vi "Teleop.vi"(10 "Match Info":T1={"Autonomous Elapsed Seconds"=0.0, "TeleOp Elapsed Seconds"=0.0, "Disabled Elapsed Seconds"=0.0, "Visited Autonomous"=FALSE, "Visited TeleOp"=FALSE, "Visited Disabled"=FALSE, "Autonomous Settings"={"Autonomous Style"=enum."Independent", "VI Refnum"=refnum}}, 11 "Call Context":T2) -> ()   [LabVIEW 2017]
doc: "This VI is called for each enabled TeleOp packet received from the DS. It is typically used to read from joysticks and other inputs and update I/O or setpoints for timed control loops. It should complete and return within 20 milliseconds or risk missing DS packets."
uses:
  <vilib>/Rock Robotics/WPI/DriverStation/WPI_DriverStationDerivedRobotMode.ctl
  <vilib>/Rock Robotics/WPI/DriverStation/WPI_DriverStationMatch Info.ctl
  Framework/Robot Global Data.vi
panel:
  out "Hardware Fault":bool
  out "Temperature Fault":bool
  out "Battery Voltage Fault":bool
  out "Current Faults":bool[](array[boolean])
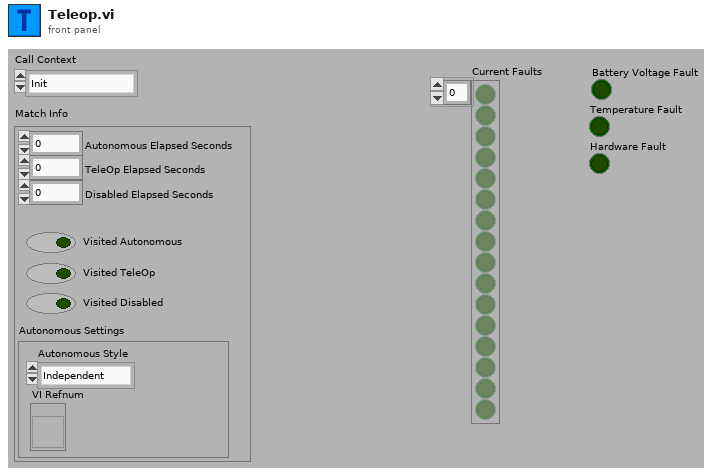
[diagram p1: front panel]
types:
  T1 = typedef "WPI_DriverStationMatch Info.ctl" = cluster{"Autonomous Elapsed Seconds":dbl, "TeleOp Elapsed Seconds":dbl, "Disabled Elapsed Seconds":dbl, "Visited Autonomous":bool, "Visited TeleOp":bool, "Visited Disabled":bool, "Autonomous Settings":cluster{"Autonomous Style":enum16{"Iterative", "Independent"}, "VI Refnum":refnum<vi>}}
  T2 = typedef "WPI_DriverStationDerivedRobotMode.ctl" = enum16{"Init", "Execute", "Stop"}
  T3 = enum16{"Linear", "Square  Root", "Square", "n^x"}
  T4 = enum16{"Normal", "Square", "Square with Rate", "Square Root", "Linear", "Exponential"}
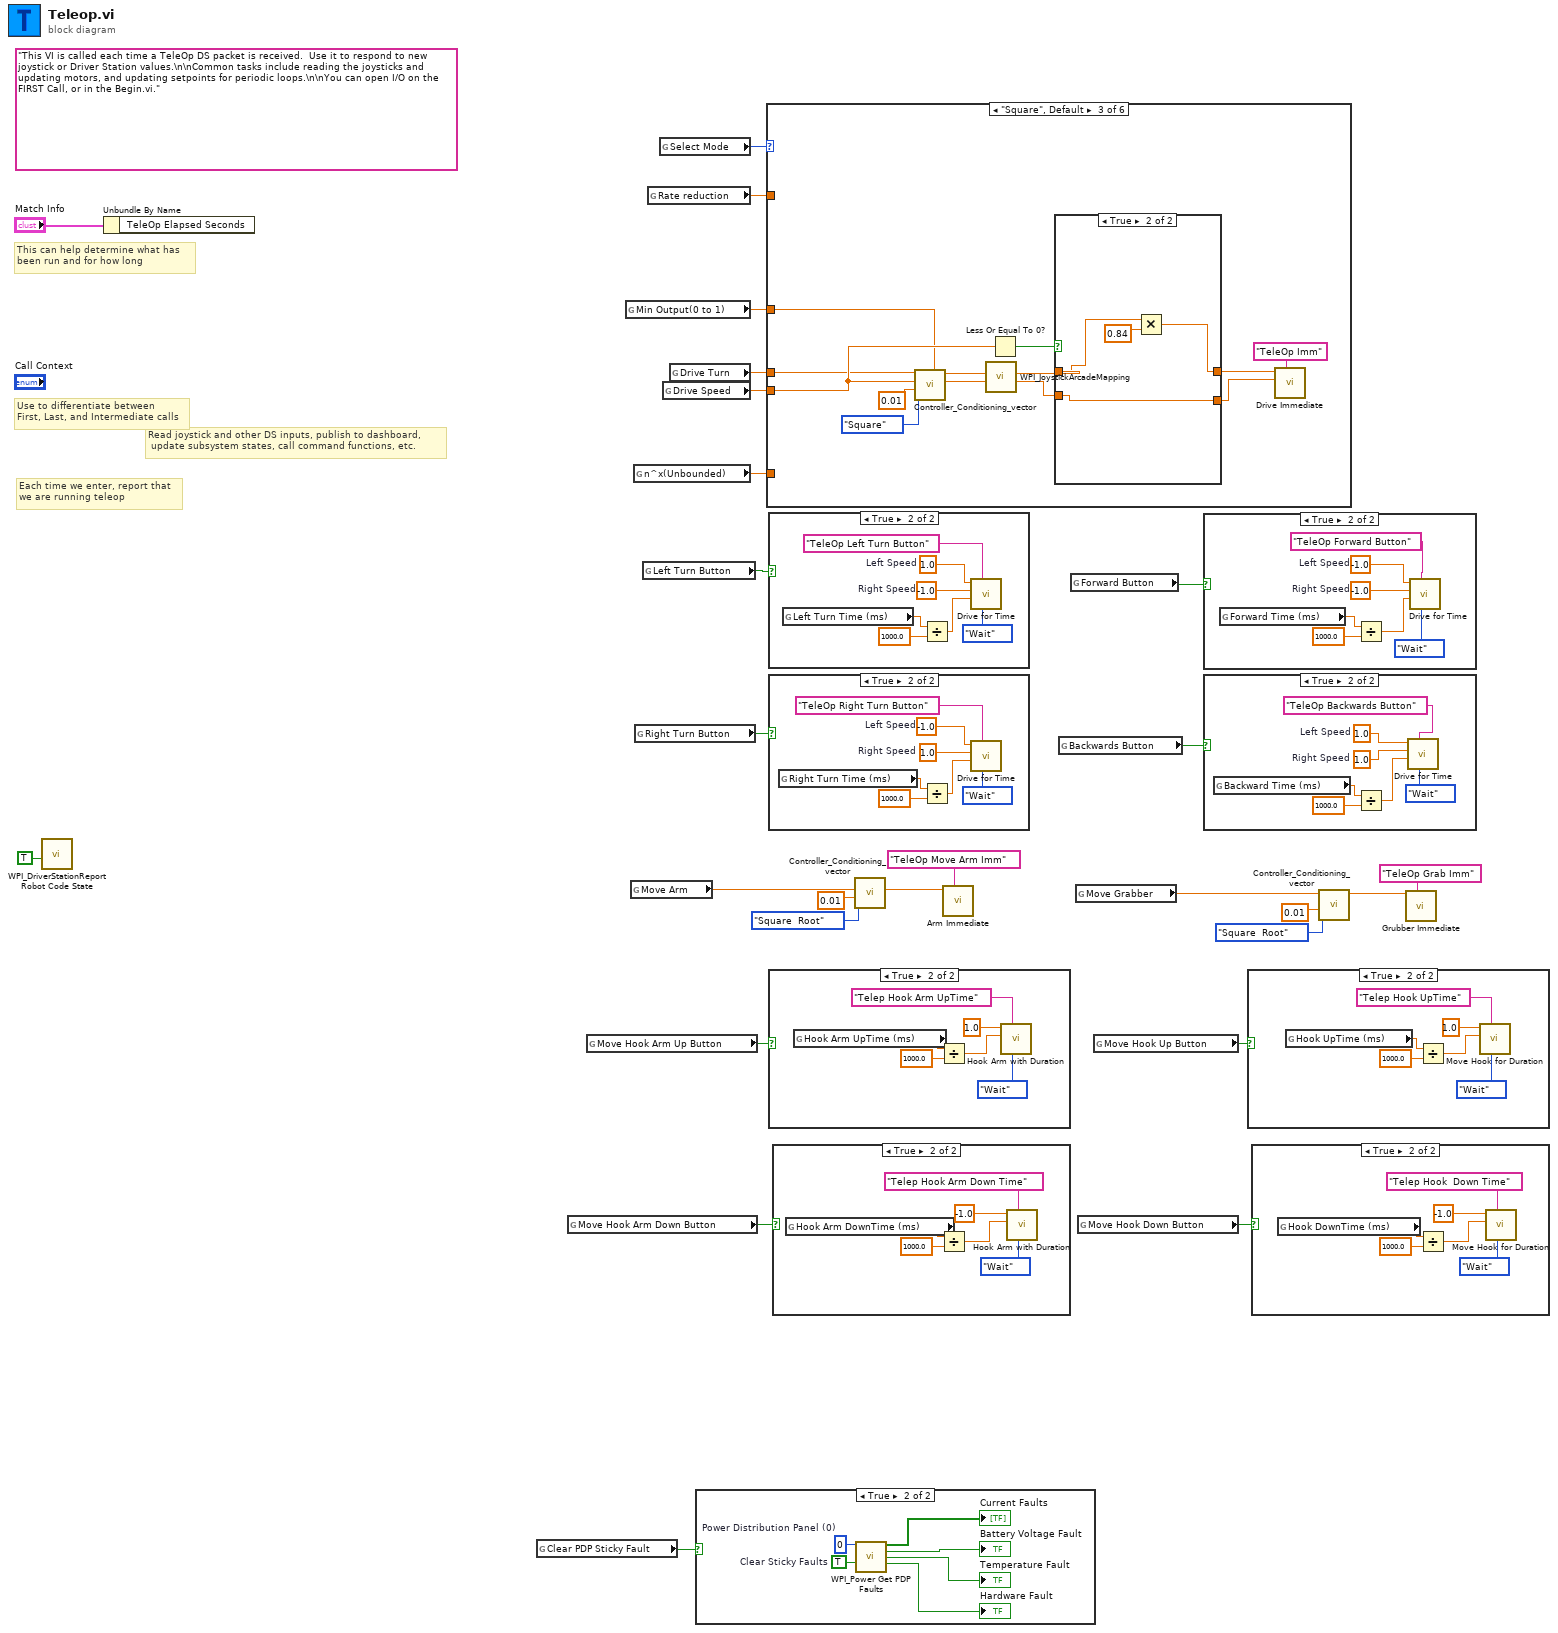
[diagram p0: block diagram]
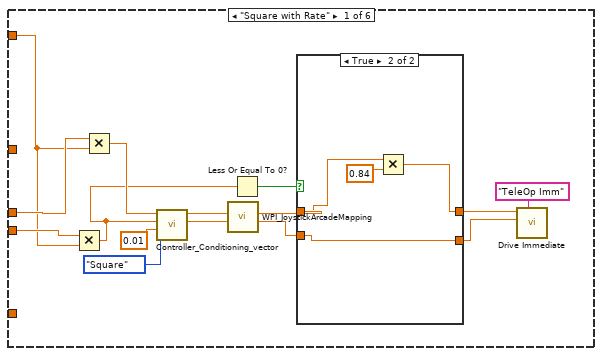
[diagram p11: hidden frame]
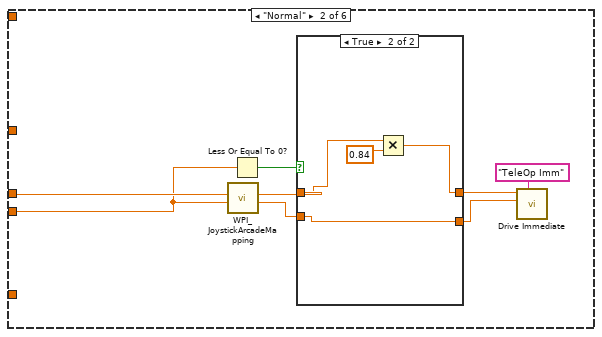
[diagram p13: hidden frame]
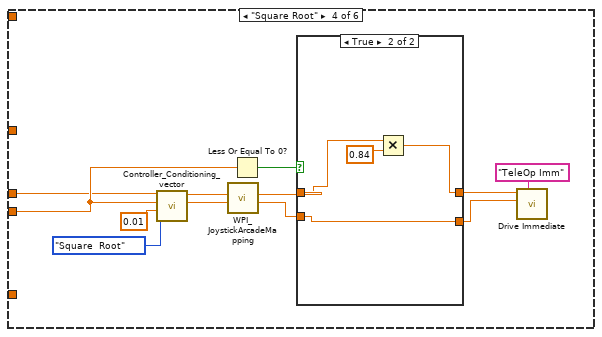
[diagram p16: hidden frame]
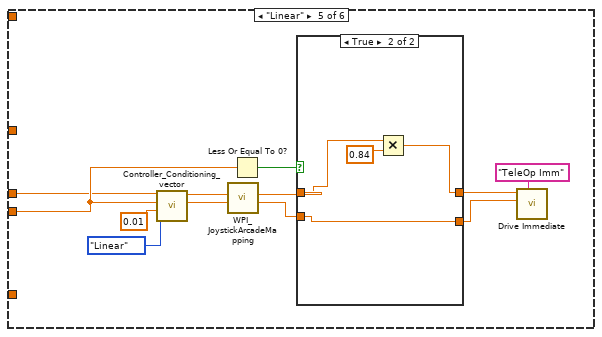
[diagram p18: hidden frame]
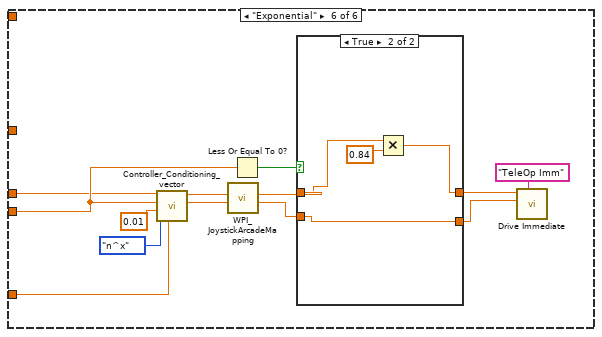
[diagram p20: hidden frame]
diagram:
  (unwired) "This VI is called each time a TeleOp DS packet is received.  Use it to respond to new joystick or Driver Station values.\n\nCommon tasks include reading the joysticks and updating motors, and updating setpoints for periodic loops.\n\nYou can open I/O on the FIRST Call, or in the Begin.vi."
  # "Read joystick and other DS inputs, publish to dashboard,\n update subsystem states, call command functions, etc."
  # "Each time we enter, report that\nwe are running teleop"
  # "Use to differentiate between\nFirst, Last, and Intermediate calls"
  # "This can help determine what has\nbeen run and for how long"
  n1 = call <vilib>:"WPI_DriverStationReport Robot Code State.vi"("TeleOp"=TRUE ("Autonomous")) -> ()  [unwired: 10 in, 1 out]
  n2 = Unbundle By Name("Match Info") -> ()  [unwired: 1 out]
  n3 = global read "Robot Global Data.vi" "Clear PDP Sticky Fault"() -> (w15:bool)
  n4 = global read "Robot Global Data.vi" "Move Hook Arm Down Button"() -> (w13:bool)
  n5 = global read "Robot Global Data.vi" "Move Hook Arm Up Button"() -> (w14:bool)
  n6 = global read "Robot Global Data.vi" "Min Output(0 to 1)"() -> (w24:dbl)
  n7 = global read "Robot Global Data.vi" "Move Arm"() -> (w17:dbl)
  n8 = global read "Robot Global Data.vi" "n^x(Unbounded)"() -> (w23:dbl)
  n9 = global read "Robot Global Data.vi" "Right Turn Button"() -> (w18:bool)
  n10 = global read "Robot Global Data.vi" "Left Turn Button"() -> (w19:bool)
  n11 = global read "Robot Global Data.vi" "Rate reduction"() -> (w22:dbl)
  n12 = global read "Robot Global Data.vi" "Select Mode"() -> (w25:T4)
  n13 = global read "Robot Global Data.vi" "Drive Speed"() -> (w20:dbl)
  n14 = global read "Robot Global Data.vi" "Drive Turn"() -> (w21:dbl)
  n15 = case shown="True" w15 {
    frame False {
    }
    frame True {
      w32 = TRUE  # Clear Sticky Faults
      w33 = u8 0  # Power Distribution Panel (0)
      n16 = call <vilib>:"WPI_Power Get PDP Faults.vi"("Power Distribution Panel (0)"=w33, "Clear Sticky Faults"=w32) -> ("Current Faults"=→"Current Faults":bool[], "Battery Voltage Fault"=→"Battery Voltage Fault":bool, "Temperature Fault"=→"Temperature Fault":bool, "Hardware Fault"=→"Hardware Fault":bool)  [unwired: 9 in, 1 out]
    }
  }
  n17 = case shown="\"Square\", Default" w25 {
    tunnel: w21 -> [w48 w56 w70 w88 w106 w125]
    tunnel: w20 -> [w47 w55 w71 w89 w107 w126]
    tunnel: w24 -> [_ _ w69 _ _ _]
    tunnel: w23 -> [_ _ _ _ _ w124]
    tunnel: w22 -> [w34 _ _ _ _ _]
    frame "Square with Rate" {
      n18 = Multiply(x=w47, y=w34) -> (x*y=w35:dbl)
      n19 = Multiply(x=w48, y=w34) -> (x*y=w36:dbl)
      n20 = call "Controller_Conditioning_vector.vi"("Enum"=T3."Square", "Dead Zone(0 to 1)"=0.01, "Y(-1 to 1)"=w35, "X(-1 to 1)"=w36) -> ("Y"=w37:dbl, "X"=w38:dbl)  [unwired: 4 in, 2 out]
      n21 = call <vilib>:"WPI_JoystickArcadeMapping.vi"("Y axis value"=w37, "X axis value"=w38) -> ("Right Motor Value"=w43:dbl, "Left Motor Value"=w44:dbl)  [unwired: 8 in]
      n22 = Less Or Equal To 0?(x=w35) -> (x <= 0?=w45:bool)
      n23 = case shown="True" w45 {
        tunnel: w44 -> [w49 w53]
        tunnel: [w49 w52] -> w42
        tunnel: w43 -> [w50 w51]
        tunnel: [w50 w51] -> w41
        frame False {
        }
        frame True {
          n24 = Multiply(x=w53, y=0.84) -> (x*y=w52:dbl)
        }
      }
      n25 = call "Drive Immediate.vi"("Description"="TeleOp Imm", "Right Setpoint"=w41, "Left Setpoint"=w42) -> ()  [unwired: 8 in, 1 out]
    }
    frame "Normal" {
      n26 = call <vilib>:"WPI_JoystickArcadeMapping.vi"("Y axis value"=w55, "X axis value"=w56) -> ("Right Motor Value"=w59:dbl, "Left Motor Value"=w60:dbl)  [unwired: 8 in]
      n27 = Less Or Equal To 0?(x=w55) -> (x <= 0?=w61:bool)
      n28 = case shown="True" w61 {
        tunnel: w60 -> [w63 w67]
        tunnel: [w63 w66] -> w58
        tunnel: w59 -> [w64 w65]
        tunnel: [w64 w65] -> w57
        frame False {
        }
        frame True {
          n29 = Multiply(x=w67, y=0.84) -> (x*y=w66:dbl)
        }
      }
      n30 = call "Drive Immediate.vi"("Description"="TeleOp Imm", "Right Setpoint"=w57, "Left Setpoint"=w58) -> ()  [unwired: 8 in, 1 out]
    }
    frame "Square", Default {
      n31 = call "Controller_Conditioning_vector.vi"("Min Output(0 to 1)"=w69, "Enum"=T3."Square", "Dead Zone(0 to 1)"=0.01, "Y(-1 to 1)"=w71, "X(-1 to 1)"=w70) -> ("Y"=w72:dbl, "X"=w73:dbl)  [unwired: 3 in, 2 out]
      n32 = call <vilib>:"WPI_JoystickArcadeMapping.vi"("Y axis value"=w72, "X axis value"=w73) -> ("Right Motor Value"=w78:dbl, "Left Motor Value"=w79:dbl)  [unwired: 8 in]
      n33 = Less Or Equal To 0?(x=w71) -> (x <= 0?=w80:bool)
      n34 = case shown="True" w80 {
        tunnel: w79 -> [w82 w86]
        tunnel: [w82 w85] -> w77
        tunnel: w78 -> [w83 w84]
        tunnel: [w83 w84] -> w76
        frame False {
        }
        frame True {
          n35 = Multiply(x=w86, y=0.84) -> (x*y=w85:dbl)
        }
      }
      n36 = call "Drive Immediate.vi"("Description"="TeleOp Imm", "Right Setpoint"=w76, "Left Setpoint"=w77) -> ()  [unwired: 8 in, 1 out]
    }
    frame "Square Root" {
      n37 = call "Controller_Conditioning_vector.vi"("Enum"=T3."Square  Root", "Dead Zone(0 to 1)"=0.01, "Y(-1 to 1)"=w89, "X(-1 to 1)"=w88) -> ("Y"=w90:dbl, "X"=w91:dbl)  [unwired: 4 in, 2 out]
      n38 = call <vilib>:"WPI_JoystickArcadeMapping.vi"("Y axis value"=w90, "X axis value"=w91) -> ("Right Motor Value"=w96:dbl, "Left Motor Value"=w97:dbl)  [unwired: 8 in]
      n39 = Less Or Equal To 0?(x=w89) -> (x <= 0?=w98:bool)
      n40 = case shown="True" w98 {
        tunnel: w97 -> [w100 w104]
        tunnel: [w100 w103] -> w95
        tunnel: w96 -> [w101 w102]
        tunnel: [w101 w102] -> w94
        frame False {
        }
        frame True {
          n41 = Multiply(x=w104, y=0.84) -> (x*y=w103:dbl)
        }
      }
      n42 = call "Drive Immediate.vi"("Description"="TeleOp Imm", "Right Setpoint"=w94, "Left Setpoint"=w95) -> ()  [unwired: 8 in, 1 out]
    }
    frame "Linear" {
      n43 = call "Controller_Conditioning_vector.vi"("Enum"=T3."Linear", "Dead Zone(0 to 1)"=0.01, "Y(-1 to 1)"=w107, "X(-1 to 1)"=w106) -> ("Y"=w108:dbl, "X"=w109:dbl)  [unwired: 4 in, 2 out]
      n44 = call <vilib>:"WPI_JoystickArcadeMapping.vi"("Y axis value"=w108, "X axis value"=w109) -> ("Right Motor Value"=w114:dbl, "Left Motor Value"=w115:dbl)  [unwired: 8 in]
      n45 = Less Or Equal To 0?(x=w107) -> (x <= 0?=w116:bool)
      n46 = case shown="True" w116 {
        tunnel: w115 -> [w118 w122]
        tunnel: [w118 w121] -> w113
        tunnel: w114 -> [w119 w120]
        tunnel: [w119 w120] -> w112
        frame False {
        }
        frame True {
          n47 = Multiply(x=w122, y=0.84) -> (x*y=w121:dbl)
        }
      }
      n48 = call "Drive Immediate.vi"("Description"="TeleOp Imm", "Right Setpoint"=w112, "Left Setpoint"=w113) -> ()  [unwired: 8 in, 1 out]
    }
    frame "Exponential" {
      n49 = call "Controller_Conditioning_vector.vi"("n^x(Unbounded)"=w124, "Enum"=T3."n^x", "Dead Zone(0 to 1)"=0.01, "Y(-1 to 1)"=w126, "X(-1 to 1)"=w125) -> ("Y"=w127:dbl, "X"=w128:dbl)  [unwired: 3 in, 2 out]
      n50 = call <vilib>:"WPI_JoystickArcadeMapping.vi"("Y axis value"=w127, "X axis value"=w128) -> ("Right Motor Value"=w133:dbl, "Left Motor Value"=w134:dbl)  [unwired: 8 in]
      n51 = Less Or Equal To 0?(x=w126) -> (x <= 0?=w135:bool)
      n52 = case shown="True" w135 {
        tunnel: w134 -> [w137 w141]
        tunnel: [w137 w140] -> w132
        tunnel: w133 -> [w138 w139]
        tunnel: [w138 w139] -> w131
        frame False {
        }
        frame True {
          n53 = Multiply(x=w141, y=0.84) -> (x*y=w140:dbl)
        }
      }
      n54 = call "Drive Immediate.vi"("Description"="TeleOp Imm", "Right Setpoint"=w131, "Left Setpoint"=w132) -> ()  [unwired: 8 in, 1 out]
    }
  }
  n55 = case shown="True" w19 {
    frame False {
    }
    frame True {
      w144 = -1.0  # Right Speed
      w143 = 1.0  # Left Speed
      n56 = global read "Robot Global Data.vi" "Left Turn Time (ms)"() -> (w148:dbl)
      n57 = Divide(x=w148, y=1000.0) -> (x/y=w149:dbl)
      n58 = call "Drive for Time.vi"("Synchronization"=enum16{"Start", "Wait"}."Wait" ("Synchronication"), "Description"="TeleOp Left Turn Button", "Seconds"=w149, "Right Speed"=w144, "Left Speed"=w143) -> ()  [unwired: 5 in, 2 out]
    }
  }
  n59 = case shown="True" w18 {
    frame False {
    }
    frame True {
      w151 = 1.0  # Right Speed
      w150 = -1.0  # Left Speed
      n60 = global read "Robot Global Data.vi" "Right Turn Time (ms)"() -> (w155:dbl)
      n61 = Divide(x=w155, y=1000.0) -> (x/y=w156:dbl)
      n62 = call "Drive for Time.vi"("Synchronization"=enum16{"Start", "Wait"}."Wait" ("Synchronication"), "Description"="TeleOp Right Turn Button", "Seconds"=w156, "Right Speed"=w151, "Left Speed"=w150) -> ()  [unwired: 5 in, 2 out]
    }
  }
  n63 = case shown="True" w14 {
    frame False {
    }
    frame True {
      n64 = global read "Robot Global Data.vi" "Hook Arm UpTime (ms)"() -> (w159:dbl)
      n65 = Divide(x=w159, y=1000.0) -> (x/y=w157:dbl)
      n66 = call "Hook Arm with Duration.vi"("Synchronization"=enum16{"Start", "Wait"}."Wait", "Description"="Telep Hook Arm UpTime", "Duration (s)"=w157, "Setpoint"=1.0) -> ()  [unwired: 7 in, 1 out]
    }
  }
  n67 = case shown="True" w13 {
    frame False {
    }
    frame True {
      n68 = global read "Robot Global Data.vi" "Hook Arm DownTime (ms)"() -> (w164:dbl)
      n69 = Divide(x=w164, y=1000.0) -> (x/y=w163:dbl)
      n70 = call "Hook Arm with Duration.vi"("Synchronization"=enum16{"Start", "Wait"}."Wait", "Description"="Telep Hook Arm Down Time", "Duration (s)"=w163, "Setpoint"=-1.0) -> ()  [unwired: 7 in, 1 out]
    }
  }
  n71 = call "Controller_Conditioning_vector.vi"("Enum"=T3."Square  Root", "Dead Zone(0 to 1)"=0.01, "Y(-1 to 1)"=w17) -> ("Y"=w8:dbl)  [unwired: 5 in, 3 out]
  n72 = call "Arm Immediate.vi"("Description"="TeleOp Move Arm Imm", "Setpoint"=w8) -> ()  [unwired: 9 in, 1 out]
  n73 = global read "Robot Global Data.vi" "Backwards Button"() -> (w12:bool)
  n74 = global read "Robot Global Data.vi" "Forward Button"() -> (w11:bool)
  n75 = global read "Robot Global Data.vi" "Move Grabber"() -> (w16:dbl)
  n76 = global read "Robot Global Data.vi" "Move Hook Down Button"() -> (w2:bool)
  n77 = global read "Robot Global Data.vi" "Move Hook Up Button"() -> (w1:bool)
  n78 = case shown="True" w11 {
    frame False {
    }
    frame True {
      w170 = -1.0  # Right Speed
      w171 = -1.0  # Left Speed
      n79 = global read "Robot Global Data.vi" "Forward Time (ms)"() -> (w172:dbl)
      n80 = Divide(x=w172, y=1000.0) -> (x/y=w169:dbl)
      n81 = call "Drive for Time.vi"("Synchronization"=enum16{"Start", "Wait"}."Wait", "Description"="TeleOp Forward Button", "Seconds"=w169, "Right Speed"=w170, "Left Speed"=w171) -> ()  [unwired: 5 in, 2 out]
    }
  }
  n82 = case shown="True" w12 {
    frame False {
    }
    frame True {
      w177 = 1.0  # Right Speed
      w178 = 1.0  # Left Speed
      n83 = global read "Robot Global Data.vi" "Backward Time (ms)"() -> (w180:dbl)
      n84 = Divide(x=w180, y=1000.0) -> (x/y=w176:dbl)
      n85 = call "Drive for Time.vi"("Synchronization"=enum16{"Start", "Wait"}."Wait", "Description"="TeleOp Backwards Button", "Seconds"=w176, "Right Speed"=w177, "Left Speed"=w178) -> ()  [unwired: 5 in, 2 out]
    }
  }
  n86 = case shown="True" w1 {
    frame False {
    }
    frame True {
      n87 = global read "Robot Global Data.vi" "Hook UpTime (ms)"() -> (w185:dbl)
      n88 = Divide(x=w185, y=1000.0) -> (x/y=w183:dbl)
      n89 = call "Move Hook for Duration.vi"("Synchronization"=enum16{"Start", "Wait"}."Wait", "Description"="Telep Hook UpTime", "Duration (s)"=w183, "Setpoint"=1.0) -> ()  [unwired: 7 in, 1 out]
    }
  }
  n90 = case shown="True" w2 {
    frame False {
    }
    frame True {
      n91 = global read "Robot Global Data.vi" "Hook DownTime (ms)"() -> (w190:dbl)
      n92 = Divide(x=w190, y=1000.0) -> (x/y=w189:dbl)
      n93 = call "Move Hook for Duration.vi"("Synchronization"=enum16{"Start", "Wait"}."Wait", "Description"="Telep Hook  Down Time", "Duration (s)"=w189, "Setpoint"=-1.0) -> ()  [unwired: 7 in, 1 out]
    }
  }
  n94 = call "Controller_Conditioning_vector.vi"("Enum"=T3."Square  Root", "Dead Zone(0 to 1)"=0.01, "X(-1 to 1)"=w16) -> ("X"=w5:dbl)  [unwired: 5 in, 3 out]
  n95 = call "Grubber Immediate.vi"("Description"="TeleOp Grab Imm", "Setpoint"=w5) -> ()  [unwired: 9 in, 1 out]
